vi "Case Structure.vi"() -> ()   [LabVIEW 2020]
panel:
  out "Numeric 2":dbl
  in  "Numeric":dbl
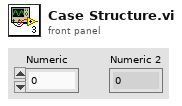
[diagram p1: front panel]
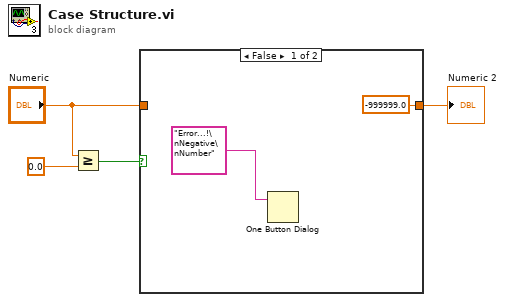
[diagram p0: block diagram]
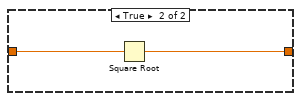
[diagram p2: hidden frame]
diagram:
  n1 = Greater Or Equal?(x="Numeric", y=0.0 ("x")) -> (x >= y?=w4:bool)
  n2 = case shown="False" w4 {
    tunnel: "Numeric" -> [_ w8]
    tunnel: [-999999.0 w7] -> w1
    frame False {
      n3 = One Button Dialog(message="Error...!\nNegative\nNumber") -> ()  [unwired: 1 in, 1 out]
    }
    frame True {
      n4 = Square Root(x=w8) -> (sqrt(x)=w7:dbl)
    }
  }
  "Numeric 2" <- w1
